vi "parameters_to_byte.vi"(8 "error in (no error)":errorcluster, 11 "UV-VIS_AVANTES in":refnum<class "UV-VIS_AVANTES.lvclass">) -> (0 "error out":errorcluster, 2 "Byte Array":u8[](array[numeric]), 3 "UV-VIS_AVANTES out":refnum<class "UV-VIS_AVANTES.lvclass">)   [LabVIEW 2020, in "UV-VIS_AVANTES.lvclass"]
uses:
  UV-VIS_AVANTES.lvclass
  UV-VIS_AVANTES.lvclass/UV-VIS_AVANTES.ctl
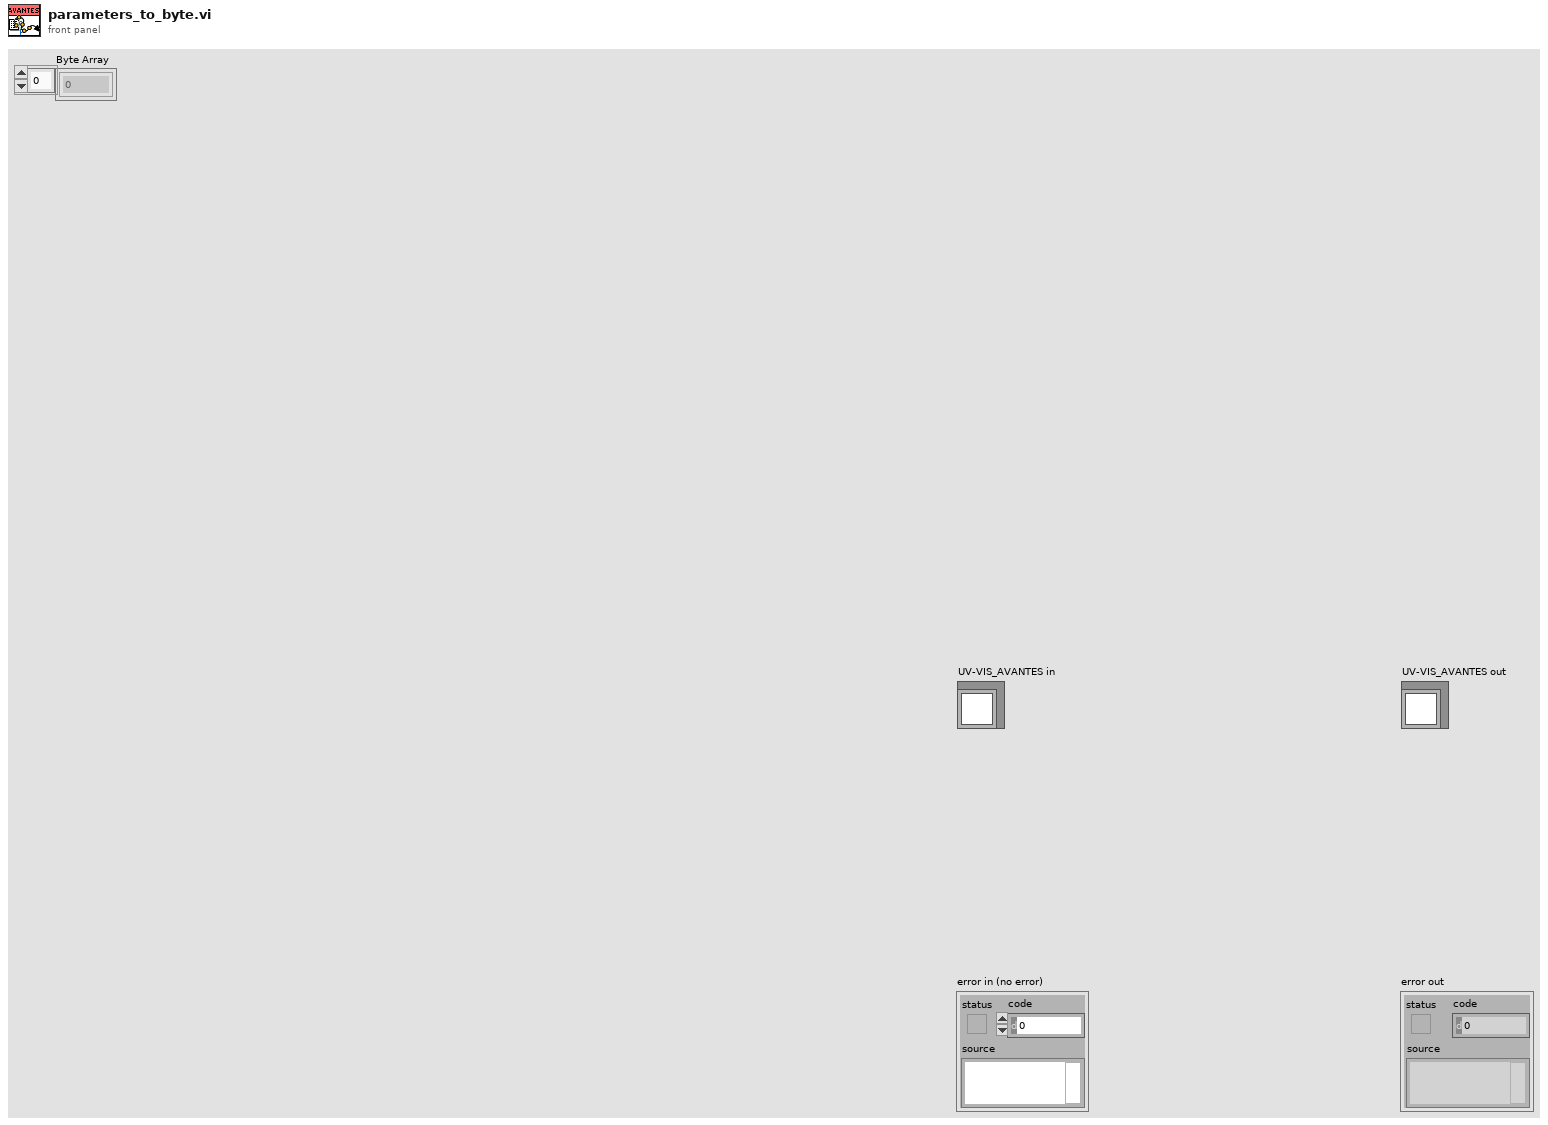
[diagram p1: front panel]
types:
  T1 = typedef "UV-VIS_AVANTES.lvclass/def_parameters.ctl" = cluster{"Len":u16, "ConfigVersion":u16, "UserFriendlyId":u8[], "DetectorType":cluster{"SensorType":u8, "NrPixels":u16, "Fit":sgl[], "NLEnable":u8, "NLCorrect":dbl[], "LowNLCounts":dbl, "HighNLCounts":dbl, "Gain":sgl[], "Reserved":sgl, "Offset":sgl[], "Extern Offset":sgl, "DefectivePixels":u16[]}, "IrradianceType":cluster{"SpectrumCalibrationType":cluster{"SmoothingType":cluster{"m_SmoothPix":u16, "SmoothModel":u8}, "CalInttime":sgl, "CalibConvers":sgl[]}, "CalibrationType":u8, "FiberDiameter":i32}, "SpectrumCalibrationType":cluster{"SmoothingType":cluster{"m_SmoothPix":u16, "SmoothModel":u8}, "CalInttime":sgl, "CalibConvers":sgl[]}, "SpectrumCorrectionType":sgl[], "StandAloneType":cluster{"StandAloneType":u8, "MeasConfigType":cluster{"StartPixel":u16, "StopPixel":u16, "IntegrationTime":sgl, "IntegrationDelay":u32, "NrAverages":u32, "DarkCorrectionType":cluster{"Enable CorDynDark":u8, "ForgetPercentage":u8}, "SmoothingType":cluster{"SmoothPix":u16, "SmoothModel":u8}, "SatDetection":u8, "TriggerType":cluster{"Trigger Mode":u8, "Trigger Source":u8, "Trigger SourceType":u8}, "ControlSettingsType":cluster{"StrobeControl":u16, "LaserDelay":u32, "LaserWidth":u32, "LaserWaveLength":sgl, "StoreToRam":u16}}, "Nmsr":i16}, "DynamicStorageType":cluster{"Nmsr":i32, "Reserved":u8[]}, "TempSensorType":sgl[], "TecControlType":cluster{"Enable":u8, "Setpoint":sgl, "Fit[NR_DAC_POL_COEF]":sgl[]}, "ProcessControlType":cluster{"AnalogLow":sgl[], "AnalogHigh":sgl[], "DigitalLow":sgl[], "DigitalHigh":sgl[]}, "EthernetSettingsType":cluster{"IpAddr":u32, "NetMask":u32, "Gateway":u32, "DhcpEnabled":u8, "TcpPort":u16, "LinkStatus":u8}, "Reserved":u8[]}
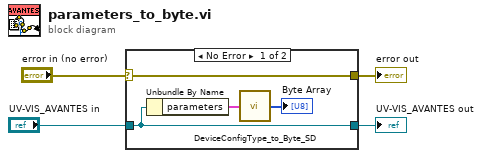
[diagram p0: block diagram]
diagram:
  n1 = case shown="No Error" "error in (no error)" {
    selector: "error in (no error)" -> [w8 w10]
    tunnel: "UV-VIS_AVANTES in" -> [w5 w9]
    tunnel: [w8 w10] -> w2
    tunnel: [w5 w9] -> w1
    frame No Error {
      n2 = Unbundle By Name(w5) -> ("parameters"=w7:T1)
      n3 = call "DeviceConfigType_to_Byte_SD.vi"("DeviceConfig"=w7) -> ("Byte Array"=→"Byte Array":u8[])  [unwired: 4 in]
    }
    frame Error {
    }
  }
  "error out" <- w2
  "UV-VIS_AVANTES out" <- w1
